vi "state & args.vi"(11 "state:args":string) -> (0 "args":string, 3 "state":string)   [LabVIEW 2021]
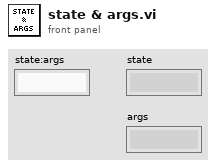
[diagram p1: front panel]
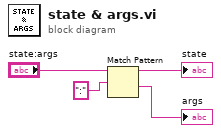
[diagram p0: block diagram]
diagram:
  n1 = Match Pattern(string="state:args", regular expression=":") -> (before substring=→"state":string, after substring=→"args":string)  [unwired: 1 in, 2 out]
